vi "PPMS2 Type.vi"(8 "error in (no error)":errorcluster, 11 "instrument.PPMS2 in":refnum<class "instrument.PPMS2.lvclass">) -> (0 "error out":errorcluster, 2 "PPMS \"Type\"":enum16{"Cryomagnetics", "QD only"}(ring), 3 "instrument.PPMS2 out":refnum<class "instrument.PPMS2.lvclass">)   [LabVIEW 2016, in "instrument.PPMS2.lvclass"]
uses:
  instrument.PPMS2.lvclass
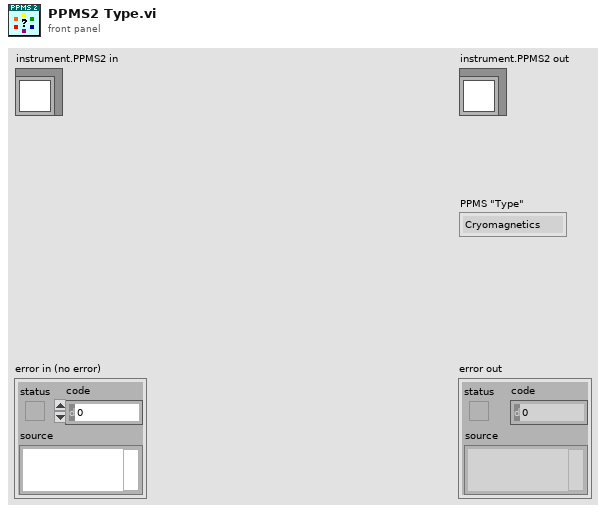
[diagram p1: front panel]
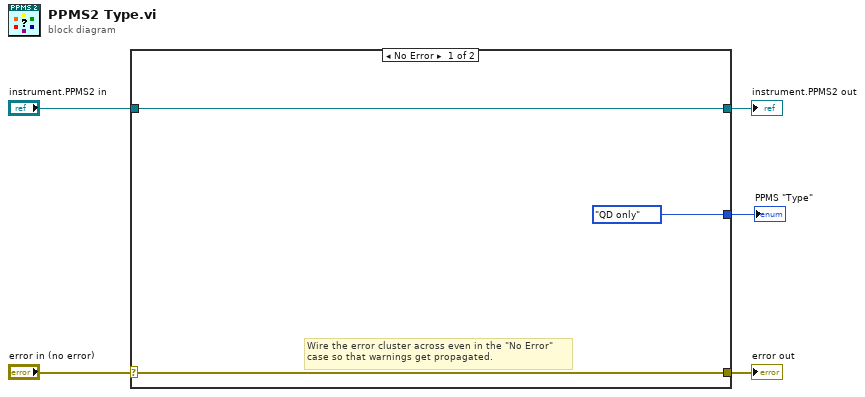
[diagram p0: block diagram]
diagram:
  n1 = case shown="No Error" "error in (no error)" {
    selector: "error in (no error)" -> [w7 w10]
    tunnel: [w7 w10] -> w4
    tunnel: [w8 w9] -> w2
    tunnel: "instrument.PPMS2 in" -> [w8 w9]
    tunnel: [enum16{"Cryomagnetics", "QD only"}."QD only" ("Enum") _] -> w1
    frame No Error {
      # "Wire the error cluster across even in the \"No Error\"\ncase so that warnings get propagated."
    }
    frame Error {
    }
  }
  "error out" <- w4
  "instrument.PPMS2 out" <- w2
  "PPMS \"Type\"" <- w1
